vi "Close TLCameraSDK.vi"(8 "error in (no error)":errorcluster, 11 "TLCameraSDK reference":refnum<k24>) -> (0 "error out":errorcluster)   [LabVIEW 2015]
uses:
  C:/code/Host/Installer/Scientific Camera Interfaces/LabVIEW/64_bit/Library_X64/Thorlabs.TSI.TLCameraInterfaces.dll
  64_bit/Library_X64/Thorlabs.TSI.TLCameraInterfaces.dll
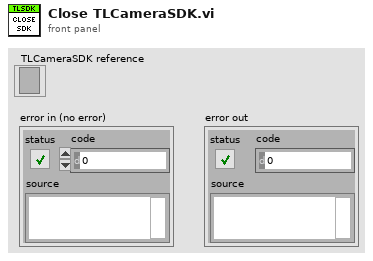
[diagram p1: front panel]
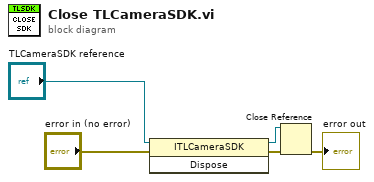
[diagram p0: block diagram]
diagram:
  n1 = invoke class="ITLCameraSDK" method="Dispose"(reference="TLCameraSDK reference", error in="error in (no error)") -> (reference out=w2:refnum<k24>, error out=w3:errorcluster)  [unwired: 1 in, 1 out]
  n2 = Close Reference(reference=w2, error in (no error)=w3) -> (error out=→"error out":errorcluster)
